vi "myRIO v1.0 Write Read SPI.vi"(8 "error in (no error)":errorcluster, 9 "Data In":u16[](array[numeric]), 10 "Channel":T1, 11 "myRIO Ref In":T2) -> (0 "error out":errorcluster, 1 "Data Out":u16[](array[numeric]), 3 "myRIO Ref Out":T2)   [LabVIEW 2021]
uses:
  <vilib>/myRIO/Common/Instrument Driver Framework/Utilities/typedefs/myRIO v1.0 Reference.ctl
  <vilib>/myRIO/Common/Instrument Driver Framework/Utilities/typedefs/Generic FPGA Reference.ctl
  <vilib>/myRIO/Common/Instrument Driver Framework/myRIO v1.0/SPI/typedefs/SPI Channels Enum.ctl
  <vilib>/myRIO/Common/Instrument Driver Framework/myRIO v1.0/SPI/typedefs/SPI Channels FPGA Reference.ctl
  <vilib>/rvi/errors/niLvFpgaAdjustHostInterfaceError.vi
  <vilib>/RVI Host/nirviSupport.llb/nirviErrorClusterFromErrorCode.vi
  <vilib>/rvi/interface/nirviReadWriteControl/nirviReadWriteControl.xnode
  <vilib>/rvi/interface/nirviMethod/nirviMethod.xnode
  <vilib>/rvi/interface/Simulation/niFpgaSimulationCallBeginRW.vi
  NiFpgaLv.dll
  <vilib>/rvi/interface/nirviMethod/StockFPGA_InlinedMethodWaitForSingleIRQ.vi
  <vilib>/FPGAPlugInAG/Dynamic/niLvFpga_WaitOnIrq_Dynamic.vi
  <vilib>/FPGAPlugInAG/Dynamic/niLvFpga_AcknowledgeIrq_Dynamic.vi
panel:
  # "This VI writes an array of data to the SPI Data Out register (SPIn.SPDO) and reads an array of data from the SPI Data In register (SPIn.SPDI) for a particular SPI channel (n). The data is written/read one value at a time. Please see Block Diagram for details."
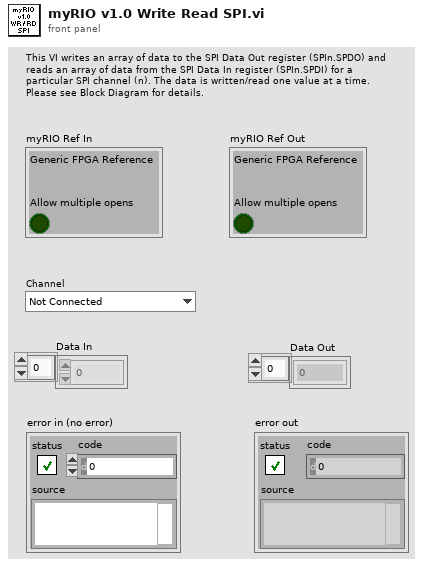
[diagram p1: front panel]
types:
  T1 = typedef "SPI Channels Enum.ctl" = enum16{"Not Connected", "A/SPI", "B/SPI", "SPI/SPI"}
  T2 = typedef "myRIO v1.0 Reference.ctl" = cluster{"Generic FPGA Reference":T3, "Allow multiple opens":bool}
  T3 = typedef "Generic FPGA Reference.ctl" = refnum<k20>
  T4 = typedef "SPI Channels FPGA Reference.ctl" = refnum<k20>
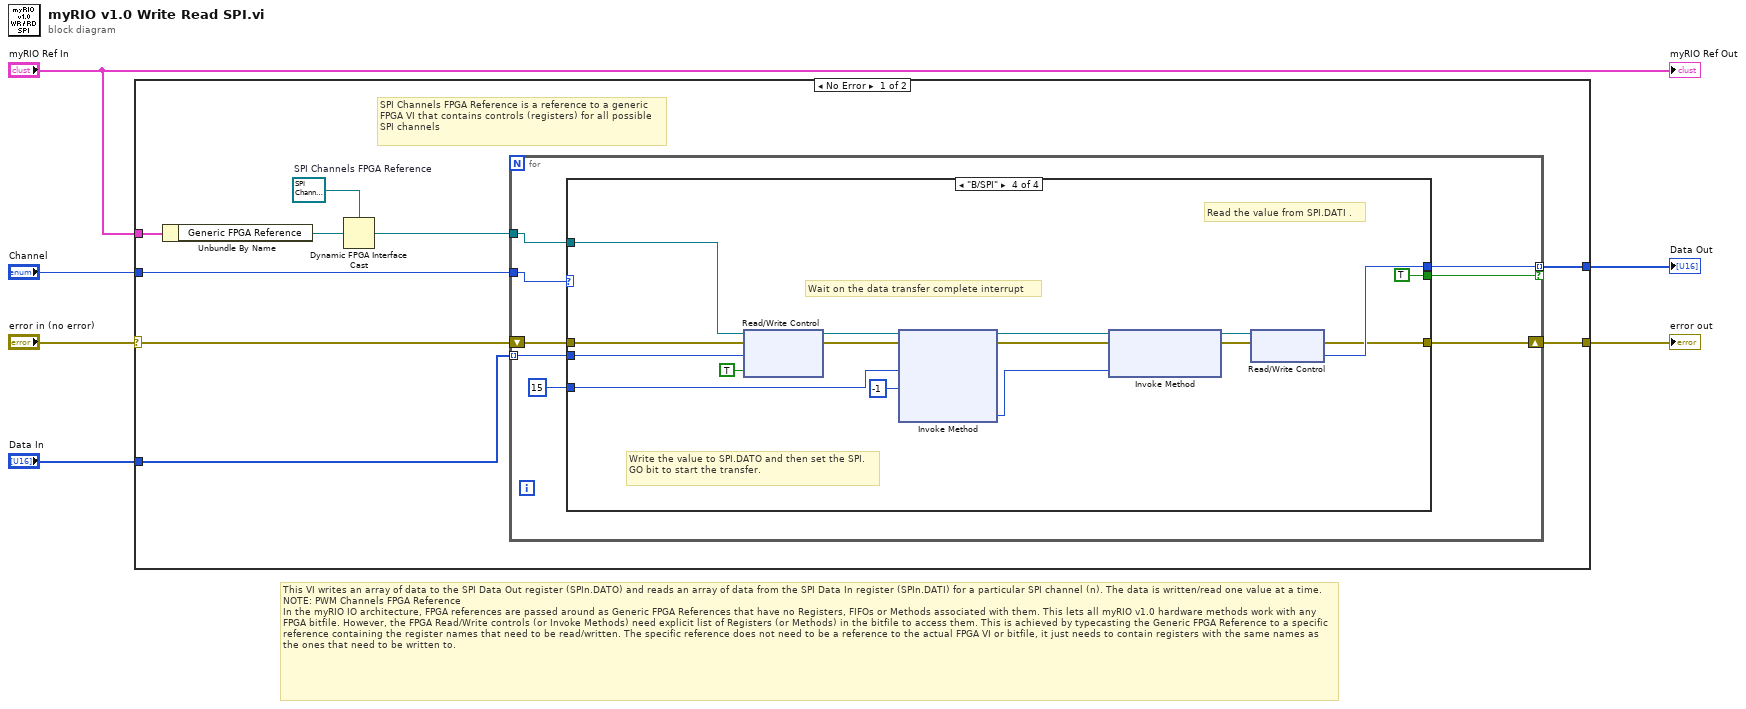
[diagram p0: block diagram]
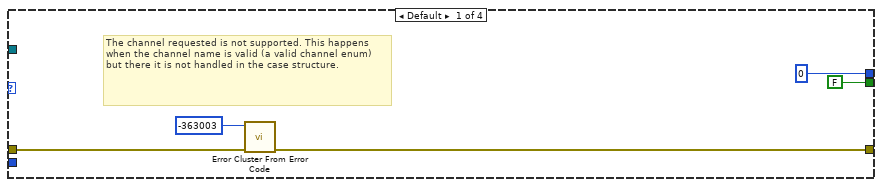
[diagram p2: hidden frame]
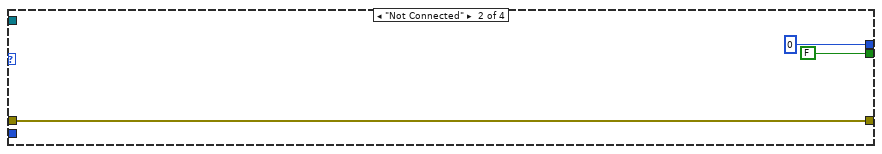
[diagram p3: hidden frame]
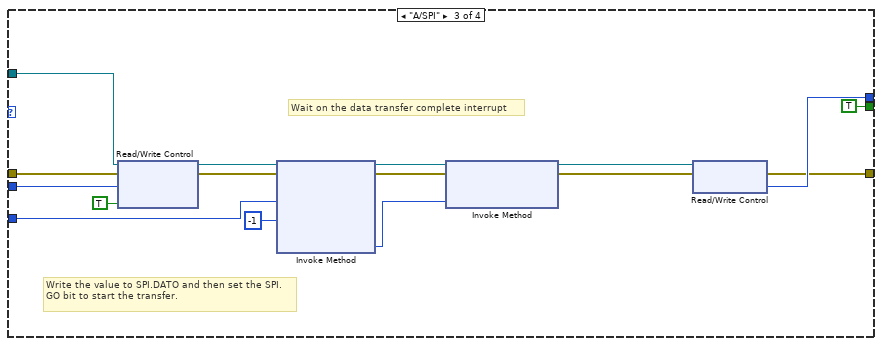
[diagram p4: hidden frame]
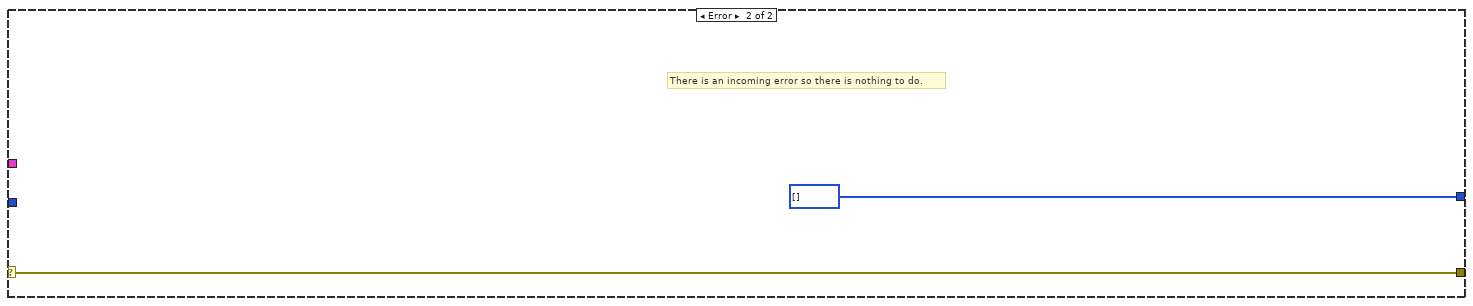
[diagram p5: hidden frame]
diagram:
  # "This VI writes an array of data to the SPI Data Out register (SPIn.DATO) and reads an array of data from the SPI Data In register (SPIn.DATI) for a particular SPI channel (n). The data is written/read one value at a time.\nNOTE: PWM Channels FPGA Reference\nIn the myRIO IO architecture, FPGA references are passed around as Generic FPGA References that have no Registers, FIFOs or Methods associated with them. This lets all myRIO v1.0 hardware methods work with any FPGA bitfile. However, the FPGA Read/Write controls (or Invoke Methods) need explicit list of Registers (or Methods) in the bitfile to access them. This is achieved by typecasting the Generic FPGA Reference to a specific reference containing the register names that need to be read/written. The specific reference does not need to be a reference to the actual FPGA VI or bitfile, it just needs to contain registers with the same names as the ones that need to be written to."
  n1 = case shown="No Error" "error in (no error)" {
    selector: "error in (no error)" -> [w8 w65]
    tunnel: [w12 u16[] [] ("t")] -> w6
    tunnel: "Channel" -> [w14 _]
    tunnel: [w13 w65] -> w4
    tunnel: "Data In" -> [w11 _]
    tunnel: "myRIO Ref In" -> [w10 _]
    frame No Error {
      w15 = T4 refnum  # SPI Channels FPGA Reference
      # "SPI Channels FPGA Reference is a reference to a generic FPGA VI that contains controls (registers) for all possible SPI channels"
      n2 = Unbundle By Name(w10) -> ("Generic FPGA Reference"=w9:T3)
      n3 = Dynamic FPGA Interface Cast(Session In=w15, Type=w9) -> (Session Out=w7:T4)
      n4 = for {
        tunnel: w7 -> [w23]
        tunnel: w14 -> [w20]
        tunnel: w11 -> [w19] mode=indexing
        tunnel: [w18] -> w12 mode=indexing if=w17
        shift-right: [w21] -> w13
        shift-left: w8 -> [w22]
        n5 = case shown="\"B/SPI\"" w20 {
          tunnel: w22 -> [w26 w31 w44 w62]
          tunnel: [w27 w31 w39 w56] -> w21
          tunnel: w23 -> [_ _ w45 w63]
          tunnel: w19 -> [_ _ w43 w61]
          tunnel: [u16 0 ("SPI1.SPDI") u16 0 ("SPI1.SPDI") w41 w58] -> w18
          tunnel: [FALSE FALSE TRUE TRUE] -> w17
          tunnel: u8 15 ("IRQ Number(s)") -> [_ _ w32 w48]
          frame Default {
            # "The channel requested is not supported. This happens when the channel name is valid (a valid channel enum) but there it is not handled in the case structure."
            n6 = call <vilib>:"Error Cluster From Error Code.vi"("error in (no error)"=w26, "error code (0)"=-363003) -> ("error out"=w27:errorcluster)  [unwired: 7 in]
          }
          frame "Not Connected" {
          }
          frame "A/SPI" {
            # "Wait on the data transfer complete interrupt"
            # "Write the value to SPI.DATO and then set the SPI.GO bit to start the transfer."
            n7 = xnode "Read/Write Control"("FPGA VI Reference In"=w45, "error in"=w44, "SPI.A.DATO"=w43, "SPI.A.GO"=TRUE) -> ("FPGA VI Reference Out"=w47:T4, "error out"=w46:errorcluster)
            n8 = xnode "Invoke Method"("FPGA VI Reference In"=w47, "error in"=w46, "IRQ Number(s)"=w32, "Timeout (ms)"=-1) -> ("FPGA VI Reference Out"=w36:T4, "error out"=w33:errorcluster, "IRQ(s) Asserted"=w34:i32)  [unwired: 1 out]
            n9 = xnode "Invoke Method"("FPGA VI Reference In"=w36, "error in"=w33, "IRQ Number(s)"=w34) -> ("FPGA VI Reference Out"=w37:T4, "error out"=w42:errorcluster)
            n10 = xnode "Read/Write Control"("FPGA VI Reference In"=w37, "error in"=w42) -> ("error out"=w39:errorcluster, "SPI.A.DATI"=w41:u16)  [unwired: 1 out]
          }
          frame "B/SPI" {
            # "Wait on the data transfer complete interrupt"
            # "Read the value from SPI.DATI ."
            # "Write the value to SPI.DATO and then set the SPI.GO bit to start the transfer."
            n11 = xnode "Read/Write Control"("FPGA VI Reference In"=w63, "error in"=w62, "SPI.B.DATO"=w61, "SPI.B.GO"=TRUE) -> ("FPGA VI Reference Out"=w49:T4, "error out"=w50:errorcluster)
            n12 = xnode "Invoke Method"("FPGA VI Reference In"=w49, "error in"=w50, "IRQ Number(s)"=w48, "Timeout (ms)"=-1) -> ("FPGA VI Reference Out"=w54:T4, "error out"=w51:errorcluster, "IRQ(s) Asserted"=w52:i32)  [unwired: 1 out]
            n13 = xnode "Invoke Method"("FPGA VI Reference In"=w54, "error in"=w51, "IRQ Number(s)"=w52) -> ("FPGA VI Reference Out"=w59:T4, "error out"=w60:errorcluster)
            n14 = xnode "Read/Write Control"("FPGA VI Reference In"=w59, "error in"=w60) -> ("error out"=w56:errorcluster, "SPI.B.DATI"=w58:u16)  [unwired: 1 out]
          }
        }
      }
    }
    frame Error {
      # "There is an incoming error so there is nothing to do."
    }
  }
  "error out" <- w4
  "Data Out" <- w6
  "myRIO Ref Out" <- "myRIO Ref In"
